vi "Reaffirm_ADAM_Outputs.vi"(3 "Reset Zeros as well":bool, 4 "Active Ch Indicies":i32[](array[numeric]), 5 "Channel Description":T1[](array[typedef]) {"Duty" format="%016b"; "D" format="%#_5g"; "C" format="%#_5g"; "B" format="%#_5g"; "A" format="%#_5g"}, 6 "Current Channel Values":dbl[](array[numeric]) format="%.2f") -> (1 "Scan Comments":string[](array[string]))   [LabVIEW 2018]
uses:
  ADAM Client/Sub VIs/ADAM Controls/Ch_description_ADAM.ctl
  ADAM Client/Sub VIs/ADAM Controls/Module_type_ADAM.ctl
  ADAM Client/Sub VIs/ADAM Controls/Function_ADAM.ctl
  ADAM Client/Sub VIs/ADAM Controls/Channel_State.ctl
  ADAM Client/Sub VIs/ADAM Controls/Calib_type_ADAM.ctl
  ADAM Client/Sub VIs/ADAM Controls/Address.ctl
  ADAM_Global.vi
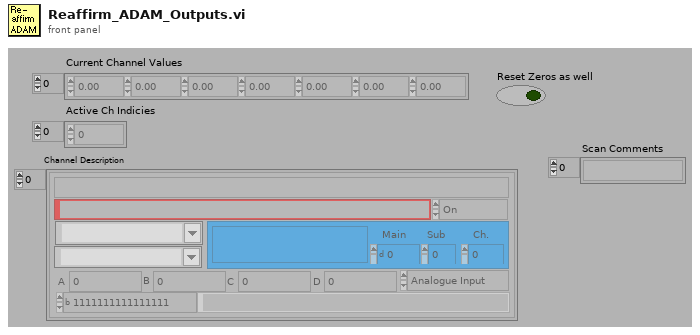
[diagram p1: front panel]
types:
  T1 = typedef "Ch_description_ADAM.ctl" = cluster{"Ch Name":string, "Type":T2, "Function":T3, "Ch State":T4, "Calibration type":T5, "A":dbl, "B":dbl, "C":dbl, "D":dbl, "Comments":string, "Address":T6, "String":string, "Duty":u16}
  T2 = typedef "Module_type_ADAM.ctl" = string
  T3 = typedef "Function_ADAM.ctl" = enum16{"Analogue Input", "Digital Input", "Event counter", "Event rate", "Analogue Output", "Digital Output", "Relay Output"}
  T4 = typedef "Channel_State.ctl" = enum16{"On", "Off", "Always On", "Always Off"}
  T5 = typedef "Calib_type_ADAM.ctl" = string
  T6 = typedef "Address.ctl" = cluster{"Main":i32, "Ch.":i32, "Sub":i32, "Port Name":string}
  T7 = typedef "Server_Control.ctl" = cluster{"Channel Name to control":string, "Channel sharing":enum16{"Channel Unshared", "Channel Shared by Rig", "Channel Shared by Group"}, "Default Value":dbl, "Client Array":string[], "Time Stamp":timestamp, "Do Not Reset":bool}
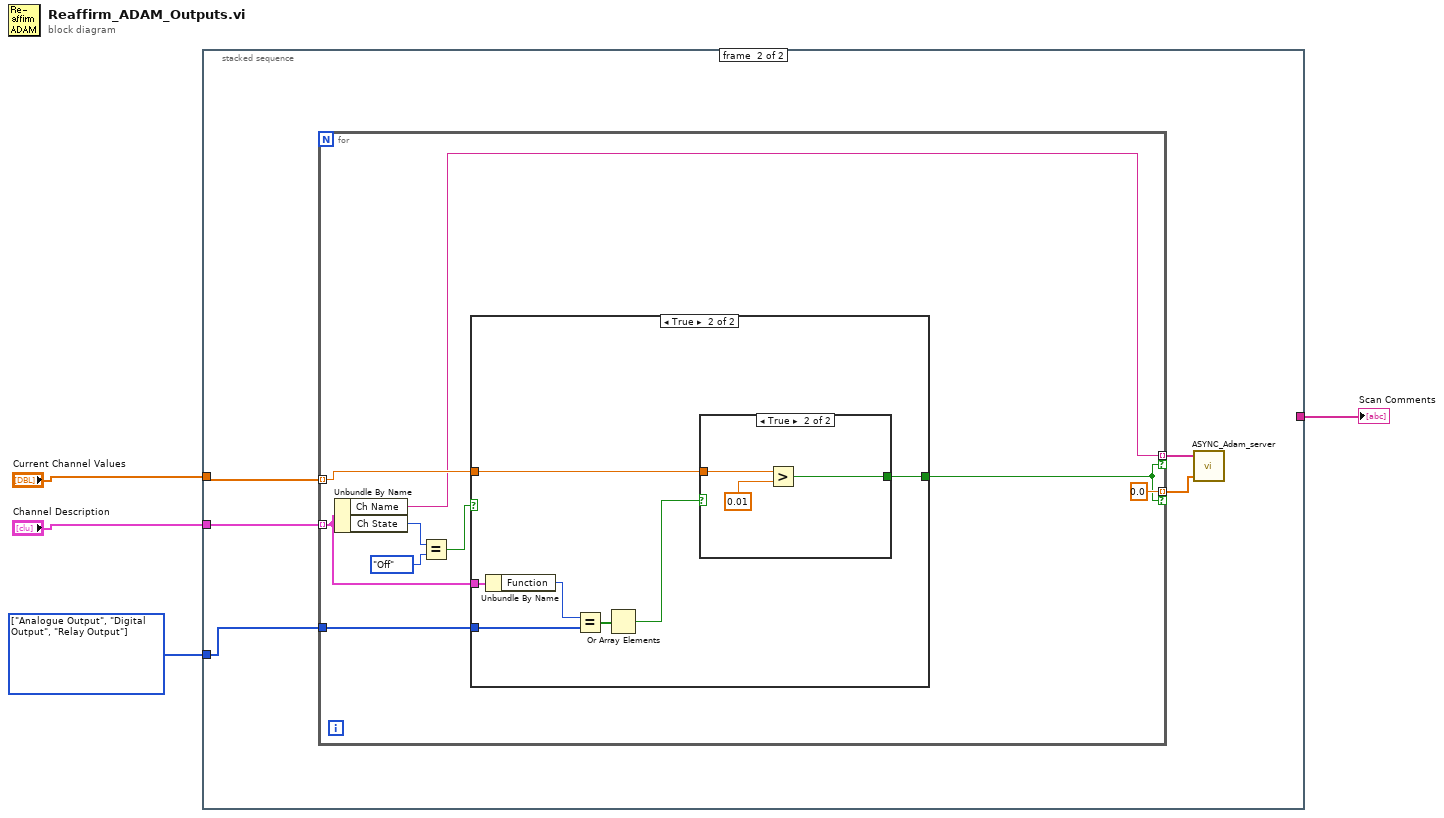
[diagram p0: block diagram]
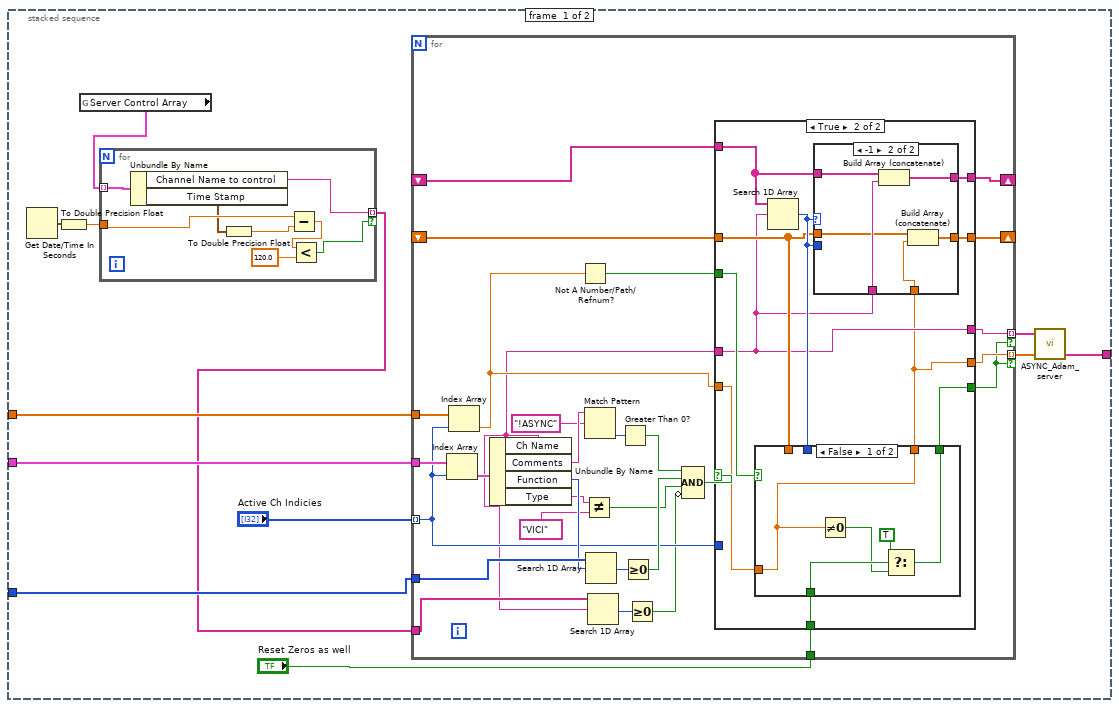
[diagram p2: hidden frame]
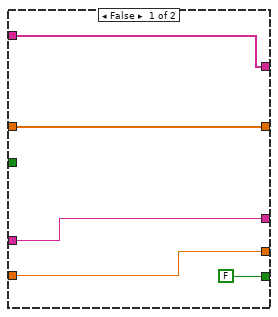
[diagram p3: hidden frame]
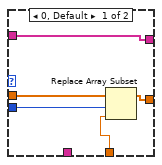
[diagram p4: hidden frame]
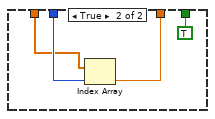
[diagram p5: hidden frame]
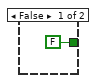
[diagram p6: hidden frame]
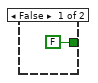
[diagram p7: hidden frame]
diagram:
  w3 = T3[] [enum."Analogue Output", enum."Digital Output", enum."Relay Output"] items=["Analogue Input", "Digital Input", "Event counter", "Event rate", "Analogue Output", "Digital Output", "Relay Output"]
  n1 = stacked-sequence {
    tunnel: "Channel Description" -> [w16 w95]
    tunnel: w3 -> [w15 w94]
    tunnel: "Current Channel Values" -> [w14 w93]
    tunnel: [w13 _] -> w1
    frame #0 {
      n2 = Get Date/Time In Seconds() -> (seconds since 1Jan1904=w11:timestamp)
      n3 = To Double Precision Float(number=w11) -> (double precision float=w10:dbl)
      n4 = global read "ADAM_Global.vi" "Server Control Array"() -> (w12:T7[])
      n5 = for {
        tunnel: w12 -> [w24] mode=indexing
        tunnel: w10 -> [w23]
        tunnel: [w18] -> w7 mode=indexing if=w17
        n6 = Unbundle By Name(w24) -> ("Channel Name to control"=w18:string, "Time Stamp"=w22:timestamp)
        n7 = To Double Precision Float(number=w22) -> (double precision float=w21:dbl)
        n8 = Subtract(x=w23, y=w21) -> (x-y=w20:dbl)
        n9 = Less?(x=w20, y=120.0) -> (x < y?=w17:bool)
      }
      n10 = for {
        tunnel: w16 -> [w44]
        tunnel: "Active Ch Indicies" -> [w42] mode=indexing
        tunnel: w15 -> [w53]
        tunnel: w14 -> [w43]
        shift-right: [w37] -> _
        shift-left: _ -> [w38]
        shift-right: [w35] -> _
        shift-left: _ -> [w36]
        tunnel: w7 -> [w32]
        tunnel: [w28] -> w9 mode=indexing if=w26
        tunnel: [w27] -> w8 mode=indexing if=w26
        tunnel: "Reset Zeros as well" -> [w25]
        n11 = Index Array(array=w44, index=w42) -> (element=w54:T1)
        n12 = Index Array(array=w43, index=w42) -> (element=w34:dbl)
        n13 = Unbundle By Name(w54) -> ("Ch Name"=w31:string, "Comments"=w51:string, "Function"=w52:T3, "Type"=w41:T2)
        n14 = Not A Number/Path/Refnum?(number/path/refnum=w34) -> (NaN/Path/Refnum?=w33:bool)
        n15 = Not Equal?(x=w41, y=T2 "VICI" ("Type")) -> (x != y?=w39:bool)
        n16 = Match Pattern(string=w51, regular expression="!ASYNC") -> (offset past match=w49:i32)  [unwired: 4 out]
        n17 = Search 1D Array(1D array=w53, element=w52) -> (index of element=w48:i32)  [unwired: 1 out]
        n18 = Search 1D Array(1D array=w32, element=w31) -> (index of element=w30:i32)  [unwired: 1 out]
        n19 = Greater Than 0?(x=w49) -> (x > 0?=w46:bool)
        n20 = Greater Or Equal To 0?(x=w48) -> (x >= 0?=w47:bool)
        n21 = Greater Or Equal To 0?(x=w30) -> (x >= 0?=w29:bool)
        n22 = Compound Arithmetic op=AND(w46, w47, w39, invert w29) -> (w45:bool)
        n23 = case shown="True" w45 {
          tunnel: w42 -> [_ _]
          tunnel: [w56 w62] -> w28
          tunnel: w31 -> [w57 w63]
          tunnel: [w57 w63] -> w27
          tunnel: w34 -> [w56 w67]
          tunnel: w38 -> [w59 w70]
          tunnel: [w59 w69] -> w37
          tunnel: w36 -> [w58 w65]
          tunnel: [w58 w68] -> w35
          tunnel: w33 -> [_ w64]
          tunnel: [FALSE w61] -> w26
          tunnel: w25 -> [_ w60]
          frame False {
          }
          frame True {
            n24 = Search 1D Array(1D array=w70, element=w63) -> (index of element=w66:i32)  [unwired: 1 out]
            n25 = case shown="False" w64 {
              tunnel: [w86 w88] -> w62
              tunnel: w67 -> [w86 _]
              tunnel: w66 -> [_ w90]
              tunnel: w65 -> [_ w89]
              tunnel: [w82 TRUE] -> w61
              tunnel: w60 -> [w85 _]
              frame False {
                n26 = Not Equal To 0?(x=w86) -> (x != 0?=w83:bool)
                n27 = Select(t=TRUE, s=w85, f=w83) -> (s? t:f=w82:bool)
              }
              frame True {
                n28 = Index Array(array=w89, index=w90) -> (element=w88:dbl)
              }
            }
            n29 = case shown="-1" w66 {
              tunnel: w70 -> [w75 w81]
              tunnel: w63 -> [_ w80]
              tunnel: [w75 w79] -> w69
              tunnel: w66 -> [w74 _]
              tunnel: w65 -> [w73 w78]
              tunnel: [w72 w76] -> w68
              tunnel: w62 -> [w71 w77]
              frame 0, Default {
                n30 = Replace Array Subset(array=w73, new element=w71, index=w74) -> (w72:dbl[])
              }
              frame -1 {
                n31 = Build Array (concatenate)(w81, w80) -> (w79:string[])
                n32 = Build Array (concatenate)(w78, w77) -> (w76:dbl[])
              }
            }
          }
        }
      }
      n33 = call "ASYNC_Adam_server.vi"("Values"=w9, "Channel Names"=w8) -> ("Scan Comments"=w13:string[])  [unwired: 1 in, 2 out]
    }
    frame #1 {
      n34 = for {
        tunnel: w95 -> [w102] mode=indexing
        tunnel: w94 -> [w101]
        tunnel: w93 -> [w100] mode=indexing
        tunnel: [w98] -> w92 mode=indexing if=w96
        tunnel: [0.0] -> w91 mode=indexing if=w96
        n35 = Unbundle By Name(w102) -> ("Ch Name"=w98:string, "Ch State"=w103:T4)
        n36 = Equal?(x=w103, y=Channel_State."Off" ("Ch State")) -> (x = y?=w99:bool)
        n37 = case shown="True" w99 {
          tunnel: w102 -> [_ w112]
          tunnel: w101 -> [_ w110]
          tunnel: w100 -> [_ w108]
          tunnel: [FALSE w106] -> w96
          frame False {
          }
          frame True {
            n38 = Unbundle By Name(w112) -> ("Function"=w111:T3)
            n39 = Equal?(x=w111, y=w110) -> (x = y?=w109:bool[])
            n40 = Or Array Elements(Boolean array=w109) -> (logical OR=w107:bool)
            n41 = case shown="True" w107 {
              tunnel: w108 -> [_ w115]
              tunnel: [FALSE w114] -> w106
              frame False {
              }
              frame True {
                n42 = Greater?(x=w115, y=0.01) -> (0:w114:bool)
              }
            }
          }
        }
      }
      n43 = call "ASYNC_Adam_server.vi"("Values"=w91, "Channel Names"=w92) -> ()  [unwired: 1 in, 3 out]
    }
  }
  "Scan Comments" <- w1
